vi "Print Graph Image.vi"(6 "Cell ID":string="s/n", 8 "Graph Reference":refnum<vi>, 9 "Sample":string="TestDesc", 10 "Project":string="TestDesc", 11 "DataPath":path) -> (0 "error out":errorcluster)   [LabVIEW 2009]
uses:
  <vilib>/Utility/NIReport.llb/NI_report.lvclass
  <vilib>/Utility/NIReport.llb/HTML Report Image Alignment.ctl
  <vilib>/Utility/NIReport.llb/NI_ReportGenerationCore.lvlib
panel:
  in  "Case Constant\n(See Context Help)":bool
  in  "Orientation":u16(ring) items=["portrait", "landscape"]
  out "ErrMsg":string
  in  "Report Type":enum16{"Standard Report", "HTML"}(ring)
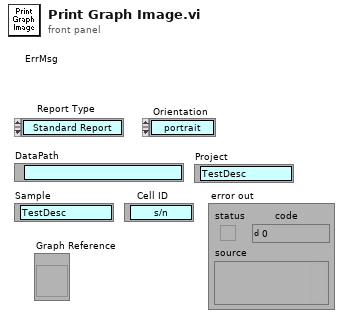
[diagram p1: front panel]
types:
  T1 = cluster{"top":dbl, "left":dbl, "right":dbl, "bottom":dbl}
  T2 = cluster{"charset (-1)":i16, "weight (-1)":i16, "name":string, "size":string}
  T3 = cluster{"Italic":enum16{"Italic Unchanged", "Italic On", "Italic Off"}, "Strike Through":enum16{"Strike Through Unchanged", "Strike Through On", "Strike Through Off"}, "Underline":enum16{"Underline Unchanged", "Underline On", "Underline Off"}, "Bold":enum16{"Bold Unchanged", "Bold On", "Bold Off"}}
  T4 = typedef "NI_ReportGenerationCore.lvlib/HTML Report Image Alignment.ctl" = enum16{"(default)", "LEFT", "RIGHT", "TOP", "TEXTTOP", "MIDDLE", "ABSMIDDLE", "BASELINE", "BOTTOM", "ABSBOTTOM"}
  T5 = enum16{"Standard Report", "HTML", "Word", "Excel"}
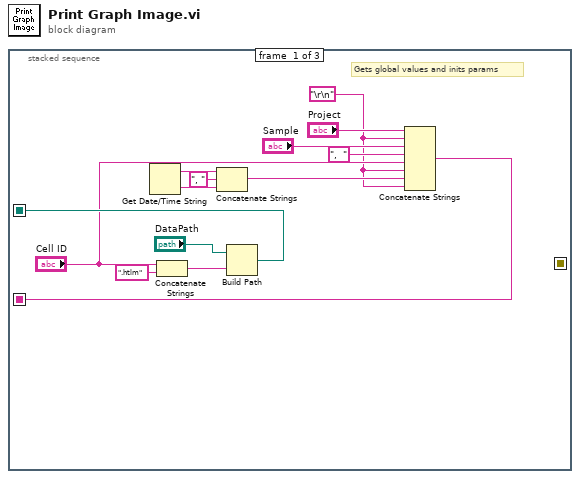
[diagram p0: block diagram]
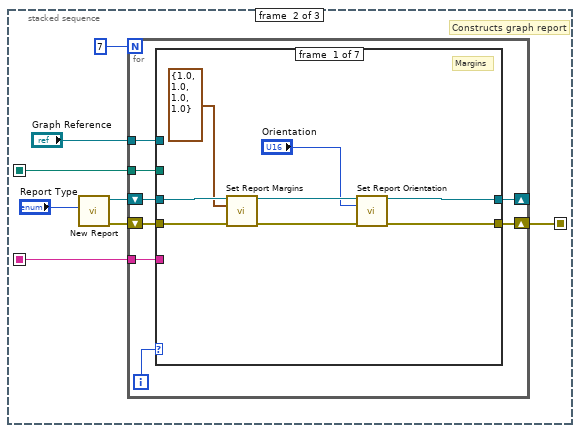
[diagram p2: hidden frame]
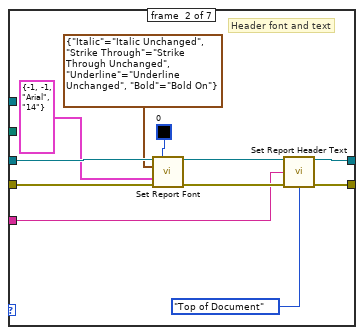
[diagram p3: hidden frame]
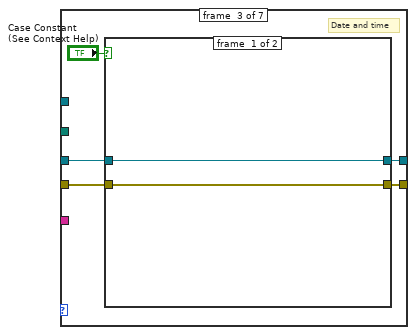
[diagram p4: hidden frame]
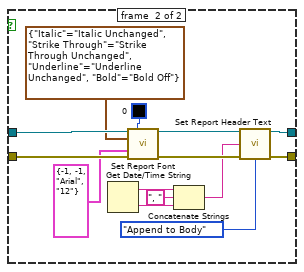
[diagram p5: hidden frame]
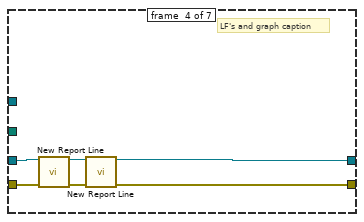
[diagram p6: hidden frame]
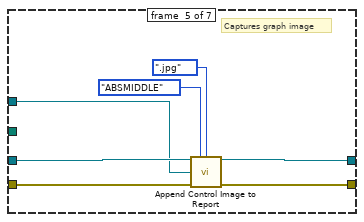
[diagram p7: hidden frame]
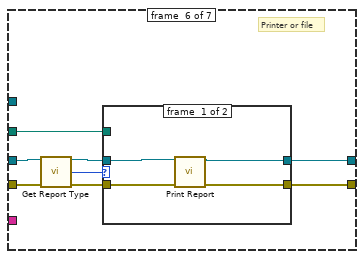
[diagram p8: hidden frame]
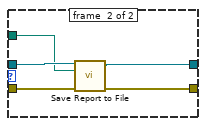
[diagram p9: hidden frame]
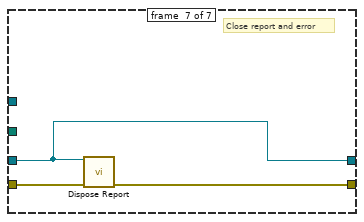
[diagram p10: hidden frame]
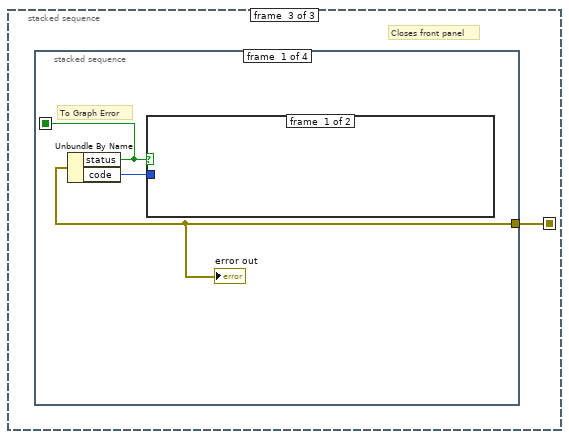
[diagram p11: hidden frame]
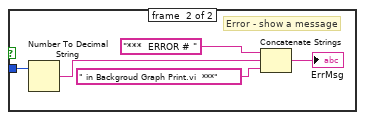
[diagram p12: hidden frame]
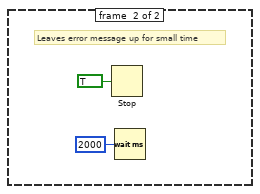
[diagram p14: hidden frame]
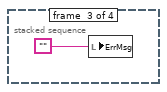
[diagram p15: hidden frame]
diagram:
  n1 = stacked-sequence {
    seq-local: [w7 _ _] -> [_ w18 _]
    seq-local: [w12 _ _] -> [_ w17 _]
    seq-local: [_ w16 _] -> [_ _ w104]
    frame #0 {
      w1 = "\r\n"
      # "Gets global values and inits params"
      n2 = Get Date/Time String() -> (date string=w10:string, time string=w9:string)  [unwired: 3 in]
      n3 = Concatenate Strings("Cell ID", ".htlm" ("string")) -> (w13:string)
      n4 = Concatenate Strings(w10, ", " ("string"), w9) -> (w2:string)
      n5 = Build Path(base path="DataPath", name or relative path=w13) -> (appended path=w12:path)
      n6 = Concatenate Strings("Project", w1, "Sample", ",  " ("string"), "Cell ID", w1, w2, w1) -> (w7:string)
    }
    frame #1 {
      # "Constructs graph report"
      n7 = call <vilib>:"New Report.vi"("report type"="Report Type") -> ("report out"=w20:refnum<class "NI_report.lvclass">, "error out"=w21:errorcluster)  [unwired: 13 in]
      n8 = for {
        N: 7 -> [_]
        shift-right: [w26] -> _
        shift-left: w20 -> [w28]
        shift-right: [w27] -> w16
        shift-left: w21 -> [w29]
        tunnel: w18 -> [w25]
        tunnel: w17 -> [w24]
        tunnel: "Graph Reference" -> [w23]
        i -> [w30]
        n9 = case shown="0, Default" w30 {
          tunnel: w29 -> [w38 w49 w54 w76 w83 w89 w103]
          tunnel: w28 -> [w37 w48 w53 w75 w81 w88 w102]
          tunnel: [w33 w42 w52 w72 w80 w90 w102] -> w26
          tunnel: [w32 w41 w51 w71 w82 w91 w101] -> w27
          tunnel: w25 -> [_ w39 _ _ _ _ _]
          tunnel: w24 -> [_ _ _ _ _ w84 _]
          tunnel: w23 -> [_ _ _ _ w77 _ _]
          frame #0 {
            # "Margins"
            n10 = call-dynamic "Set Report Margins.vi"("report in"=w37, "margins (1.00)"=T1 {"top"=1.0, "left"=1.0, "right"=1.0, "bottom"=1.0}, "error in (no error)"=w38) -> ("report out"=w35:refnum<class "NI_report.lvclass">, "error out"=w34:errorcluster)  [unwired: 10 in, 1 out]
            n11 = call-dynamic "Set Report Orientation.vi"("report in"=w35, "orientation (portrait)"="Orientation", "error in (no error)"=w34) -> ("report out"=w33:refnum<class "NI_report.lvclass">, "error out"=w32:errorcluster)  [unwired: 11 in]
          }
          frame #1 {
            # "Header font and text"
            n12 = call-dynamic "Set Report Font.vi"("report in"=w48, "text color (unchanged)"=u32 0, "text options"=T3 {"Italic"=enum."Italic Unchanged", "Strike Through"=enum."Strike Through Unchanged", "Underline"=enum."Underline Unchanged", "Bold"=enum."Bold On"}, "font settings"=T2 {"charset (-1)"=-1, "weight (-1)"=-1, "name"="Arial", "size"="14"}, "error in (no error)"=w49) -> ("report out"=w44:refnum<class "NI_report.lvclass">, "error out"=w43:errorcluster)  [unwired: 8 in, 1 out]
            n13 = call-dynamic "Set Report Header Text.vi"("report in"=w44, "center header text"=w39, "error in (no error)"=w43, "header placement"=enum16{"Top of Document", "Append to Body"}."Top of Document") -> ("report out"=w42:refnum<class "NI_report.lvclass">, "error out"=w41:errorcluster)  [unwired: 10 in]
          }
          frame #2 {
            # "Date and time"
            n14 = case shown="True" "Case Constant\n(See Context Help)" {
              tunnel: w54 -> [w55 w70]
              tunnel: w53 -> [w56 w69]
              tunnel: [w56 w63] -> w52
              tunnel: [w55 w62] -> w51
              frame #0 {
              }
              frame #1 {
                n15 = Get Date/Time String() -> (date string=w60:string, time string=w59:string)  [unwired: 3 in]
                n16 = call-dynamic "Set Report Font.vi"("report in"=w69, "text color (unchanged)"=u32 0, "text options"=T3 {"Italic"=enum."Italic Unchanged", "Strike Through"=enum."Strike Through Unchanged", "Underline"=enum."Underline Unchanged", "Bold"=enum."Bold Off"}, "font settings"=T2 {"charset (-1)"=-1, "weight (-1)"=-1, "name"="Arial", "size"="12"}, "error in (no error)"=w70) -> ("report out"=w65:refnum<class "NI_report.lvclass">, "error out"=w64:errorcluster)  [unwired: 8 in, 1 out]
                n17 = Concatenate Strings(w60, ", " ("string"), w59) -> (w58:string)
                n18 = call-dynamic "Set Report Header Text.vi"("report in"=w65, "center header text"=w58, "error in (no error)"=w64, "header placement"=enum16{"Top of Document", "Append to Body"}."Append to Body") -> ("report out"=w63:refnum<class "NI_report.lvclass">, "error out"=w62:errorcluster)  [unwired: 10 in]
              }
            }
          }
          frame #3 {
            # "LF's and graph caption"
            n19 = call-dynamic "New Report Line.vi"("report in"=w75, "error in (no error)"=w76) -> ("report out"=w73:refnum<class "NI_report.lvclass">, "error out"=w74:errorcluster)  [unwired: 12 in]
            n20 = call-dynamic "New Report Line.vi"("report in"=w73, "error in (no error)"=w74) -> ("report out"=w72:refnum<class "NI_report.lvclass">, "error out"=w71:errorcluster)  [unwired: 12 in]
          }
          frame #4 {
            # "Captures graph image"
            n21 = call-dynamic "Append Control Image to Report.vi"("report in"=w81, "alignment (default)"=HTML_Report_Image_Alignment."ABSMIDDLE", "image file type (.jpg)"=enum16{".jpg", ".png"}.".jpg" ("image file type(.jpg)"), "ctrl reference"=w77, "error in (no error)"=w83) -> ("report out"=w80:refnum<class "NI_report.lvclass">, "error out"=w82:errorcluster)  [unwired: 7 in, 2 out]
          }
          frame #5 {
            # "Printer or file"
            n22 = call-dynamic "Get Report Type.vi"("report in"=w88, "error in (no error)"=w89) -> ("report out"=w87:refnum<class "NI_report.lvclass">, "report type"=w85:T5, "error out"=w86:errorcluster)  [unwired: 11 in]
            n23 = case shown="\"HTML\"" w85 {
              tunnel: w87 -> [w94 w100]
              tunnel: w86 -> [w95 w99]
              tunnel: [w92 w98] -> w91
              tunnel: [w93 w97] -> w90
              tunnel: w84 -> [_ w96]
              frame #0 {
                n24 = call-dynamic "Print Report.vi"("report in"=w94, "error in (no error)"=w95) -> ("report out"=w93:refnum<class "NI_report.lvclass">, "error out"=w92:errorcluster)  [unwired: 12 in]
              }
              frame #1 {
                n25 = call-dynamic "Save Report to File.vi"("report in"=w100, "report file path"=w96, "error in (no error)"=w99) -> ("report out"=w97:refnum<class "NI_report.lvclass">, "error out"=w98:errorcluster)  [unwired: 11 in]
              }
            }
          }
          frame #6 {
            # "Close report and error"
            n26 = call-dynamic "Dispose Report.vi"("report in"=w102, "error in (no error)"=w103) -> ("error out"=w101:errorcluster)  [unwired: 13 in]
          }
        }
      }
    }
    frame #2 {
      # "Closes front panel"
      n27 = stacked-sequence {
        seq-local: [w105 _ _ _] -> [_ w113 _ _]
        tunnel: w104 -> [w107 _ _ _]
        frame #0 {
          # "To Graph Error"
          n28 = Unbundle By Name(w107) -> ("status"=w105:bool, "code"=w106:i32)
          n29 = case shown="True" w105 {
            tunnel: w106 -> [_ w111]
            frame #0 {
            }
            frame #1 {
              # "Error - show a message"
              n30 = Number To Decimal String(number=w111) -> (decimal integer string=w110:string)  [unwired: 1 in]
              n31 = Concatenate Strings("***  ERROR # " ("string"), w110, " in Backgroud Graph Print.vi  ***" ("string")) -> (→"ErrMsg":string)
            }
          }
          "error out" <- w107
        }
        frame #1 {
          n32 = case shown="True" w113 {
            frame #0 {
            }
            frame #1 {
              # "Leaves error message up for small time"
              n33 = Stop(stop? (T)=TRUE) -> ()
              n34 = Wait (ms)(milliseconds to wait=u32 2000) -> ()  [unwired: 1 out]
            }
          }
        }
        frame #2 {
          n35 = local write "ErrMsg"("") -> ()
        }
        frame #3 {
        }
      }
    }
  }
